vi "DefineColorPalette.vi"(10 "Files in":T1[](array[typedef]), 11 "FileList":refnum<vi>) -> (2 "Files out":T1[](array[typedef]))   [LabVIEW 2022 SP3]
uses:
  Curtin1_Label.ctl
panel:
  in  "Delete":bool
  in  "Clear":bool
  in  "Save":bool
  in  "Save as":bool
  in  "Apply":bool
  in  "Your Color Palettes":u16(ring) items=["Last Saved", "24 Colors", "All Black", "All Red", "klklj"]
  in  "Colors":u32[](array[colorbox])
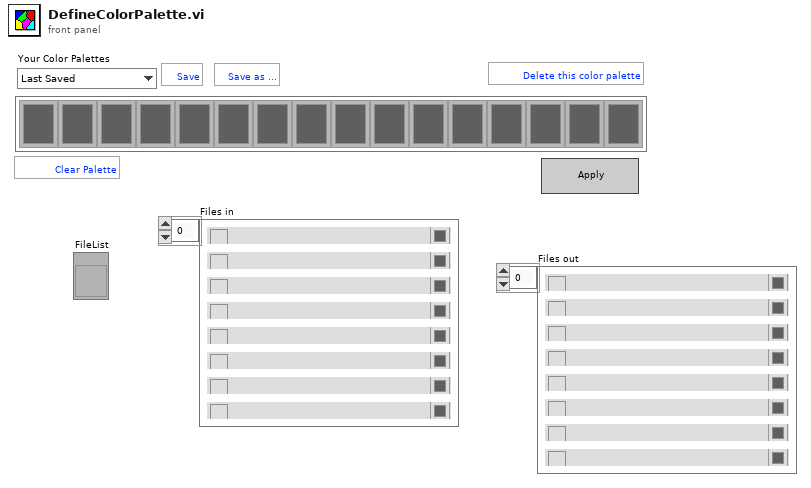
[diagram p1: front panel]
types:
  T1 = typedef "Curtin1_Label.ctl" = cluster{"Show?":bool, "Name":string, "Color":u32, "Path":path, "Show Notes":bool}
  T2 = enum16{"big-endian, network order", "native, host order", "little-endian"}
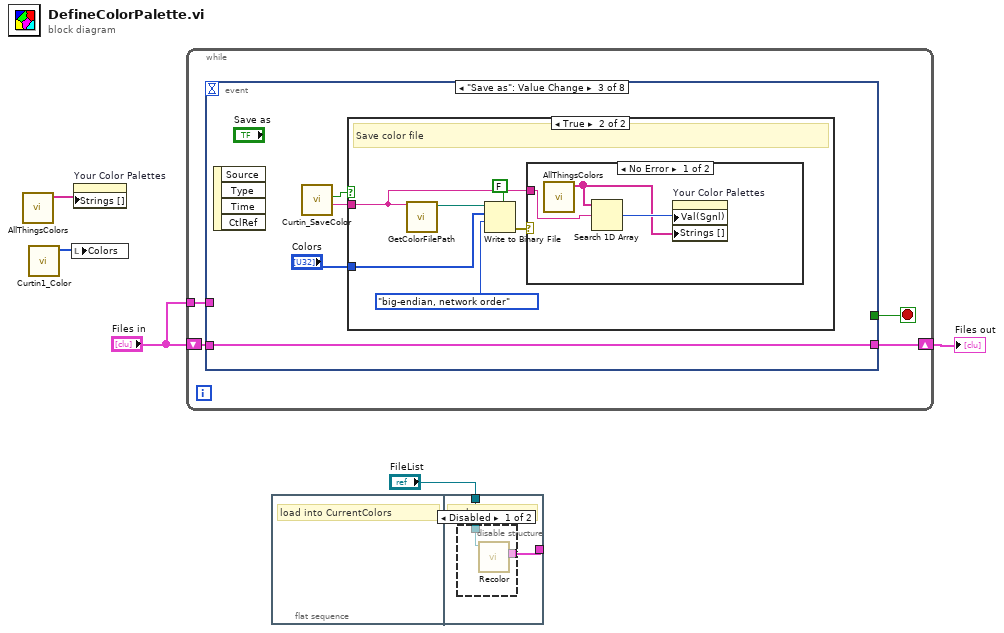
[diagram p0: block diagram]
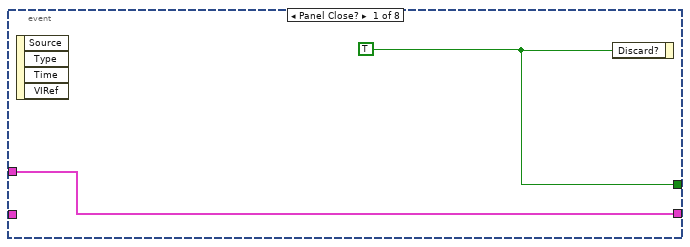
[diagram p3: hidden frame]
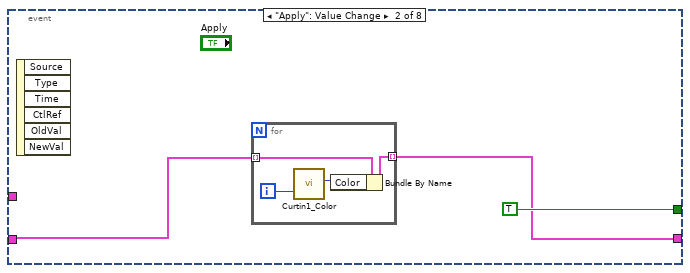
[diagram p4: hidden frame]
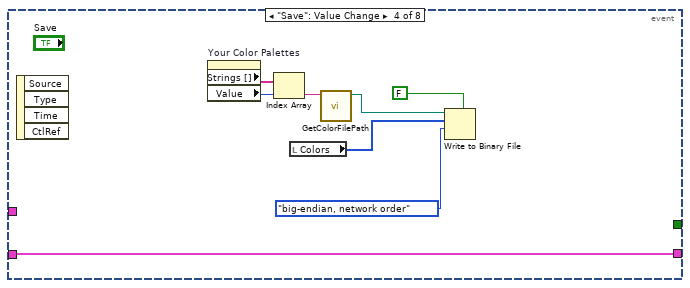
[diagram p7: hidden frame]
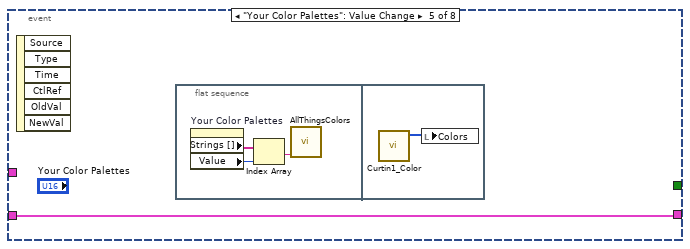
[diagram p8: hidden frame]
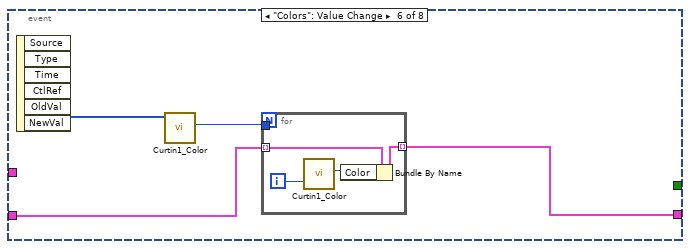
[diagram p9: hidden frame]
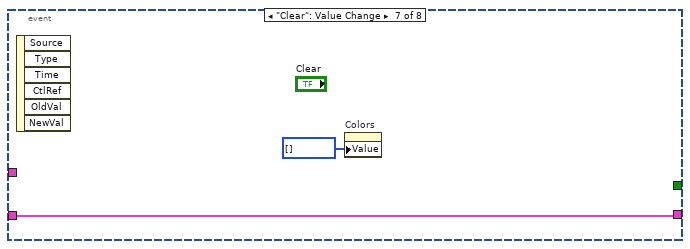
[diagram p10: hidden frame]
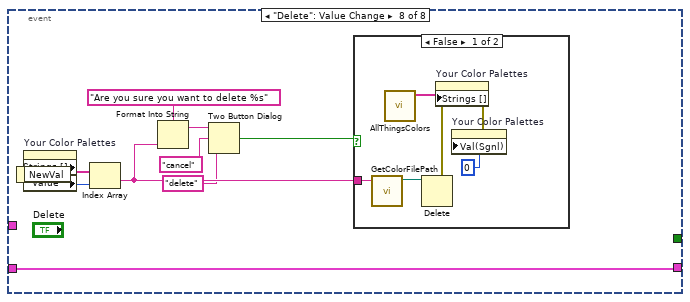
[diagram p11: hidden frame]
diagram:
  n1 = call "AllThingsColors.vi"() -> ("Possible Colors"=w5:string[])  [unwired: 11 in]
  n2 = call "Curtin1_Color.vi"() -> ("Color palette"=w1:u32[])  [unwired: 10 in, 1 out]
  n3 = local write "Colors"(w1) -> ()
  n4 = property on="Your Color Palettes" class="Ring (strict)"("Strings []"=w5) -> ()  [unwired: 2 in, 2 out]
  n5 = while {
    shift-right: [w8] -> w4
    shift-left: "Files in" -> [w7]
    tunnel: "Files in" -> [w6]
    stop <- w9 stop-if-true
    n6 = event shown="[2] \"Save as\": Value Change" {
      selector: _ -> [_ _ _ _ _ _ _ _]
      dyn-events: _ -> [_ _ _ _ _ _ _ _]
      timeout: _ -> [_ _ _ _ _ _ _ _]
      tunnel: [w11 TRUE ("Discard?") _ _ _ _ _ _] -> w9
      tunnel: [w10 w13 w20 w39 w40 w46 w54 w63] -> w8
      tunnel: w7 -> [_ w12 w20 w39 w40 w47 w54 w63]
      tunnel: w6 -> [w10 _ _ _ _ _ _ _]
      event Panel Close? {
        w11 = TRUE ("Discard?")
        n7 = event-data() -> ()  [unwired: 1 in, 4 out]
        n8 = event-data("Discard?"=w11) -> ()  [unwired: 1 in, 1 out]
      }
      event "Apply": Value Change {
        n9 = event-data() -> ()  [unwired: 1 in, 6 out]
        n10 = for {
          tunnel: w12 -> [w18] mode=indexing
          tunnel: [w17] -> w13 mode=indexing
          i -> [w16]
          n11 = call "Curtin1_Color.vi"("Offset"=w16) -> ("New color"=w15:u32)  [unwired: 9 in, 1 out]
          n12 = Bundle By Name(cluster=w18, "Color"=w15) -> (w17:T1)
        }
      }
      event "Save as": Value Change {
        n13 = event-data() -> ()  [unwired: 1 in, 4 out]
        n14 = call "Curtin_SaveColor.vi"() -> ("New Color"=w22:string, "Good?"=w21:bool)  [unwired: 10 in]
        n15 = case shown="True" w21 {
          tunnel: w22 -> [_ w23]
          tunnel: "Colors" -> [_ w25]
          frame False {
          }
          frame True {
            # "Save color file"
            n16 = call "GetColorFilePath.vi"("String"=w23) -> ("path"=w24:path)  [unwired: 9 in, 1 out]
            n17 = Write to Binary File(file (use dialog)=w24, data=w25, 5:FALSE ("prepend array or string size? (T)"), 9:T2."big-endian, network order" ("byte order (0:big-endian, network order)")) -> (error out=w26:errorcluster)  [unwired: 2 in, 2 out]
            n18 = case shown="No Error" w26 {
              tunnel: w23 -> [w31 _]
              frame No Error {
                n19 = call "AllThingsColors.vi"() -> ("Possible Colors"=w29:string[])  [unwired: 11 in]
                n20 = Search 1D Array(1D array=w29, element=w31) -> (index of element=w30:i32)  [unwired: 1 in]
                n21 = property on="Your Color Palettes" class="Ring (strict)"("Val(Sgnl)"=w30, "Strings []"=w29) -> ()  [unwired: 2 in, 2 out]
              }
              frame Error {
              }
            }
          }
        }
      }
      event "Save": Value Change {
        n22 = event-data() -> ()  [unwired: 1 in, 4 out]
        n23 = property on="Your Color Palettes" class="Ring (strict)"() -> ("Strings []"=w33:string[], "Value"=w34:u16)  [unwired: 2 in, 2 out]
        n24 = Index Array(array=w33, index=w34) -> (element=w32:string)
        n25 = local read "Colors"() -> (w35:u32[])
        n26 = call "GetColorFilePath.vi"("String"=w32) -> ("path"=w36:path)  [unwired: 9 in, 1 out]
        n27 = Write to Binary File(file (use dialog)=w36, data=w35, 5:FALSE ("prepend array or string size? (T)"), 9:T2."big-endian, network order" ("byte order (0:big-endian, network order)")) -> ()  [unwired: 2 in, 3 out]
      }
      event "Your Color Palettes": Value Change {
        n28 = event-data() -> ()  [unwired: 1 in, 6 out]
        n29 = flat-sequence {
          frame #0 {
            n30 = property on="Your Color Palettes" class="Ring (strict)"() -> ("Strings []"=w42:string[], "Value"=w41:u16)  [unwired: 2 in, 2 out]
            n31 = Index Array(array=w42, index=w41) -> (element=w43:string)
            n32 = call "AllThingsColors.vi"("Choice"=w43) -> ()  [unwired: 10 in, 1 out]
          }
          frame #1 {
            n33 = call "Curtin1_Color.vi"() -> ("Color palette"=w44:u32[])  [unwired: 10 in, 1 out]
            n34 = local write "Colors"(w44) -> ()
          }
        }
      }
      event "Colors": Value Change {
        n35 = event-data() -> ("NewVal"=w48:u32[])  [unwired: 1 in, 5 out]
        n36 = call "Curtin1_Color.vi"("Color"=w48) -> ("New color"=w45:u32)  [unwired: 9 in, 1 out]
        n37 = for {
          tunnel: w47 -> [w52] mode=indexing
          tunnel: [w51] -> w46 mode=indexing
          tunnel: w45 -> [_]
          i -> [w50]
          n38 = call "Curtin1_Color.vi"("Offset"=w50) -> ("New color"=w49:u32)  [unwired: 9 in, 1 out]
          n39 = Bundle By Name(cluster=w52, "Color"=w49) -> (w51:T1)
        }
      }
      event "Clear": Value Change {
        n40 = event-data() -> ()  [unwired: 1 in, 6 out]
        n41 = property on="Colors" class="Arr (strict)"("Value"=u32[] [] ("Colors")) -> ()  [unwired: 2 in, 2 out]
      }
      event "Delete": Value Change {
        n42 = event-data() -> ()  [unwired: 1 in, 1 out]
        n43 = property on="Your Color Palettes" class="Ring (strict)"() -> ("Strings []"=w61:string[], "Value"=w62:u16)  [unwired: 2 in, 2 out]
        n44 = Index Array(array=w61, index=w62) -> (element=w59:string)
        n45 = Format Into String(format string="Are you sure you want to delete %s", w59) -> (resulting string=w58:string)  [unwired: 2 in, 1 out]
        n46 = Two Button Dialog(message=w58, 1:"delete" ("F button name (\"Cancel\")"), 2:"cancel" ("T button name (\"OK\")")) -> (T button?=w55:bool)
        n47 = case shown="False" w55 {
          tunnel: w59 -> [w69 _]
          frame False {
            n48 = call "GetColorFilePath.vi"("String"=w69) -> ("path"=w68:path)  [unwired: 9 in, 1 out]
            n49 = call "AllThingsColors.vi"() -> ("Possible Colors"=w66:string[])  [unwired: 11 in]
            n50 = Delete(path (use dialog)=w68) -> (error out=w65:errorcluster)  [unwired: 4 in, 2 out]
            n51 = property on="Your Color Palettes" class="Ring (strict)"(error in=w65, "Strings []"=w66) -> (error out=w64:errorcluster)  [unwired: 1 in, 1 out]
            n52 = property on="Your Color Palettes" class="Ring (strict)"(error in=w64, "Val(Sgnl)"=0) -> ()  [unwired: 1 in, 2 out]
          }
          frame True {
          }
        }
      }
    }
  }
  "Files out" <- w4
  n53 = flat-sequence {
    tunnel: "FileList" -> [w71]
    tunnel: [w70] -> _
    frame #0 {
      # "load into CurrentColors"
    }
    frame #1 {
      # "replot"
      n54 = disable-structure shown="Disabled" {
        disable-tunnel: w71 -> [w73 _]
        disable-tunnel: [w72 _] -> w70
        frame Disabled {
          n55 = call "Recolor.vi"("Array in"=w73) -> ("Files"=w72:T1[])  [unwired: 10 in]
        }
        frame Enabled {
        }
      }
    }
  }
